vi "View one AI param scada1.vi"(5 "Sensors refs":refnum<vi>[](array[refnum]), 6 "OPC UA.Client refnum":T2, 7 "AI Descr":string[][](array[string]), 8 "error in (no error)":errorcluster, 9 "AIP":dbl[][](array[numeric]), 10 "AI_State":T3[](array[typedef]), 11 "AITable":dbl[](array[numeric]) format="%#.0f") -> (0 "error out":errorcluster)   [LabVIEW 2019, in "Inputs.lvlib"]
uses:
  Inputs.lvlib
  Ctl/Parameter State.ctl
  <vilib>/OPCUA/controls/OPC UA Client Refnum.ctl
  Ctl/View one AI param State.ctl
  <vilib>/Utility/miscctls.llb/LVRowAndColumnUnsignedTypeDef.ctl
  Ctl/AIParamColumns.ctl
  <vilib>/OPCUA/controls/NodeId.ctl
  <vilib>/OPCUA/client/Multiple Write Variant.vi
  <vilib>/OPCUA/NI OPC UA Client.lvlib
  OPC/OPC addons.lvlib
panel:
  in  "Tab Control":T1(tab)
  in  "input_register_min":dbl min=-32768.0 max=65535.0 step=1.0 format="%#.0f"
  in  "input_register_max":dbl min=-32768.0 max=65535.0 step=1.0 format="%#.0f"
  in  "input_pv_min":dbl format="%#.1f"
  in  "input_pv_max":dbl format="%#.1f"
  in  "instrument_gain":dbl min=-32768.0 max=65535.0 step=1.0 format="%#.0f"
  in  "instrument_offset":dbl format="%#.3f"
  in  "sensor num":i32
  in  "instrument_min_offset":dbl min=-32768.0 max=65535.0 step=1.0 format="%#.0f"
  in  "time_const":dbl min=-32768.0 max=65535.0 step=1.0 format="%#.0f"
  in  "fcode_full":string="кгс/см2"
  out "AI_1":dbl format="%#.1f"
  in  "Param":i32(listbox) caption="Параметры"
  in  "d":dbl min=-32768.0 max=65535.0 step=1.0 format="%#.0f"
  in  "instrument_max_offset":dbl min=-32768.0 max=65535.0 step=1.0 format="%#.0f"
  out "units":string="кгс/см2"
  in  "instrument_range_max":dbl format="%#.1f"
  in  "process_range_max":dbl format="%#.1f"
  in  "process_high_acd":dbl format="%#.1f"
  in  "process_high_alr":dbl format="%#.1f"
  in  "process_low_alr":dbl format="%#.1f"
  in  "process_low_acd":dbl format="%#.1f"
  in  "process_range_min":dbl format="%#.1f"
  in  "instrument_range_min":dbl format="%#.1f"
  # "Настройка пределов"
  # "верхнийний предел датчика"
  # "верхний предел достоверных показаний"
  # "верхний аварийный предел"
  # "верхний предупредительный предел"
  # "нижний предупредительный предел"
  # "нижний аварийный предел"
  # "нижний предел достоверных показаний"
  # "нижний предел датчика"
  # "Y"
  # "значение сигнала максимум (Ymax)"
  # "значение сигнала минимум (Ymin)"
  # "X"
  # "входной регистр минимум (Xmin)"
  # "входной регистр максимум (Xmax)"
  # "Y"
  # "массштабирование"
  # "смещение"
  # "X"
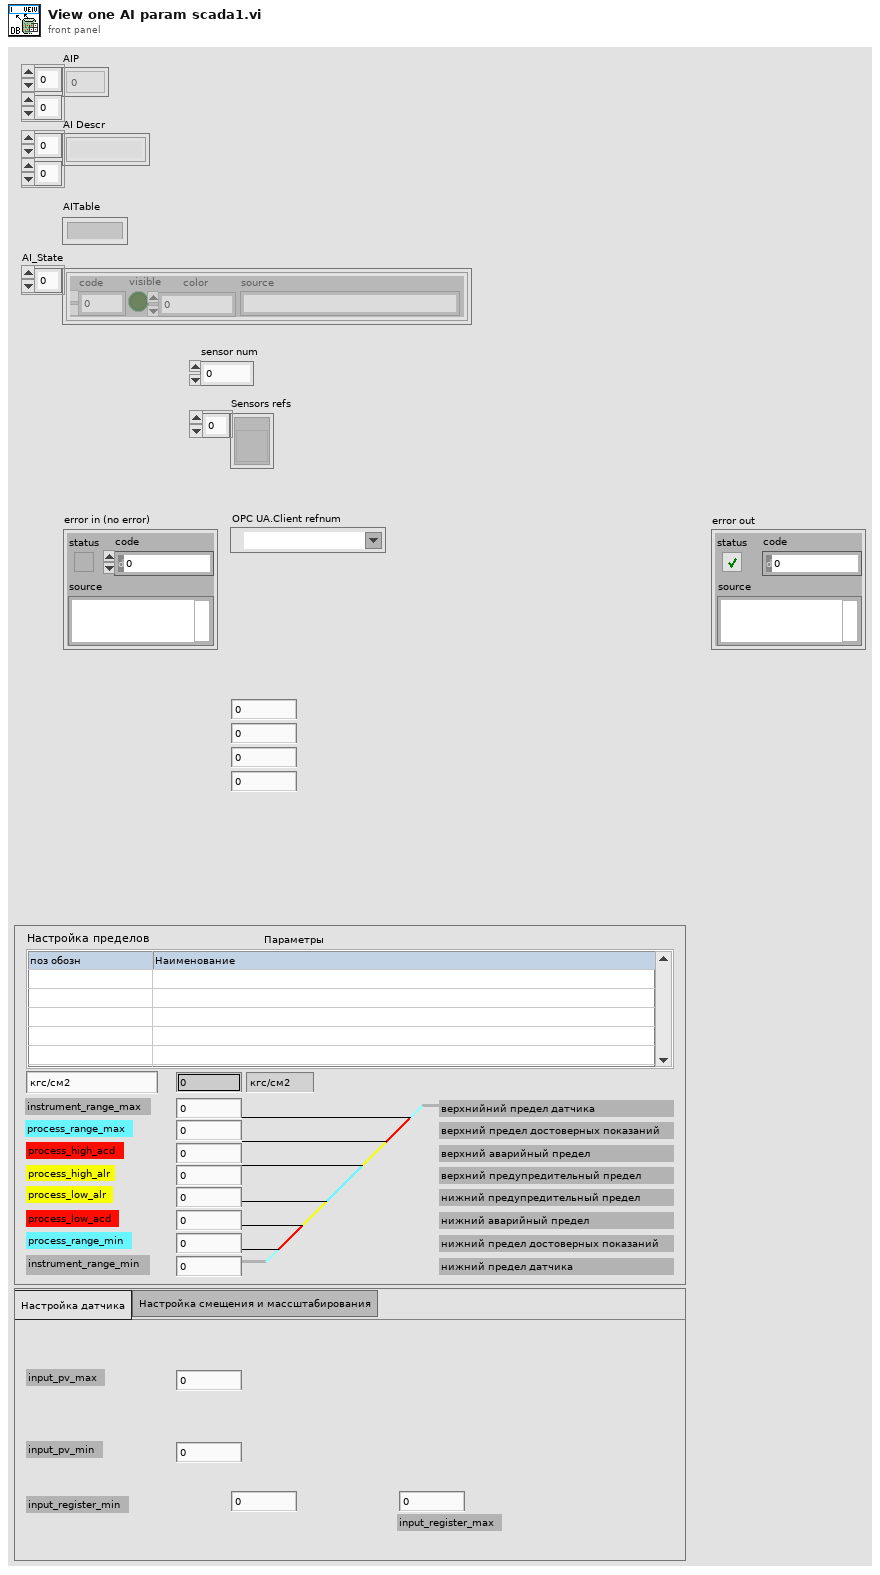
[diagram p1: front panel]
types:
  T1 = enum32{"Настройка датчика", "Настройка смещения и массштабирования"}
  T2 = typedef "OPC UA Client Refnum.ctl" = refnum<k21>
  T3 = typedef "Inputs.lvlib/Parameter State.ctl" = cluster{"code":i32, "visible":bool, "color":u32, "source":string}
  T4 = typedef "Inputs.lvlib/View one AI param State.ctl" = enum16{"init", "change sensor", "wait changes", "write parameters"}
  T5 = typedef "LVRowAndColumnUnsignedTypeDef.ctl" = cluster{"Row":u32, "Column":u32}
  T6 = typedef "NodeId.ctl" = string
  T7 = typedef "Inputs.lvlib/AIParamColumns.ctl" = enum16{"instrument_gain", "instrument_offset", "time_const", "instrument_min_offset", "instrument_range_min", "process_range_min", "process_low_acd", "process_low_alr", "process_high_alr", "process_high_acd", "process_range_max", "instrument_range_max", "instrument_max_offset", "d", "input_register_min", "input_register_max", "input_pv_min", "input_pv_max", "module_fcode_full", "control_channel_num", "ip_adress", "fcode", "fcodef", "fcode_full", "fname", "process_units"}
  T8 = typedef "Write Variant Request.ctl" = cluster{"node ID":T6, "value":variant, "timestamp (current time)":timestamp, "node status":T9}
  T9 = typedef "Write Status.ctl" = u32
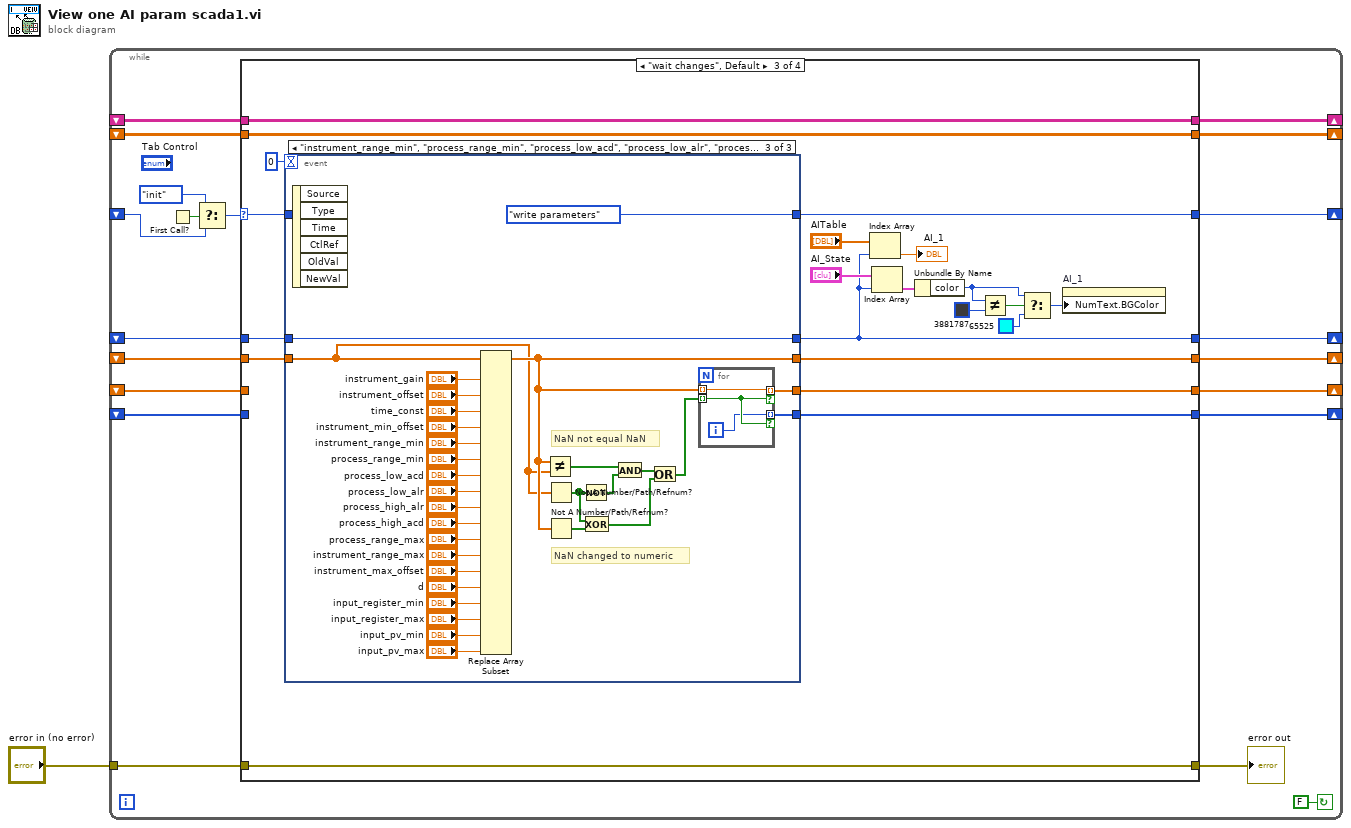
[diagram p0: block diagram]
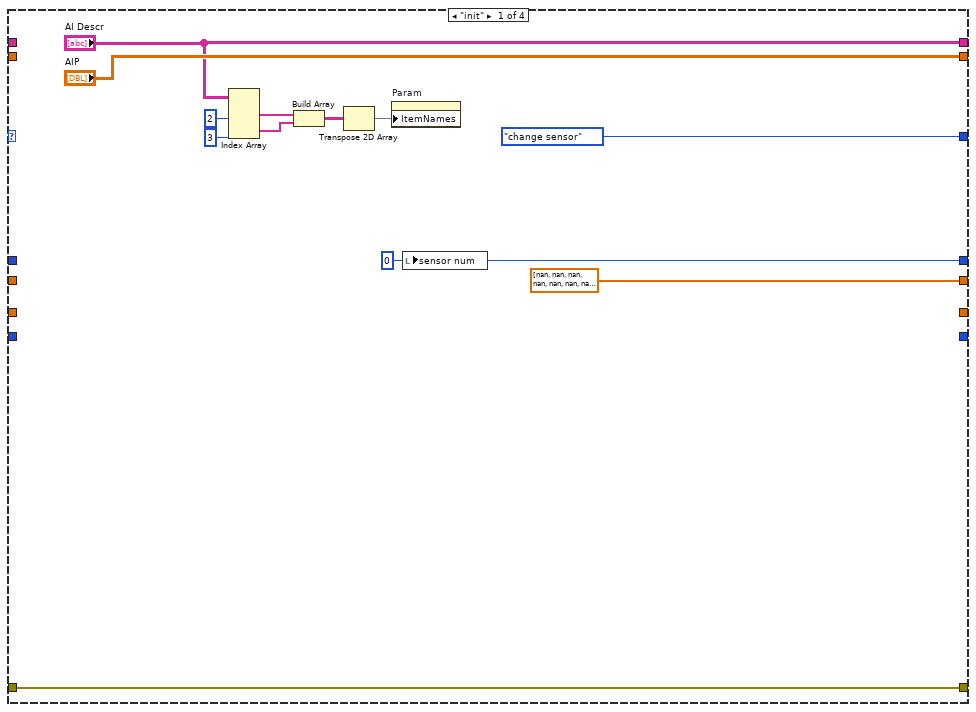
[diagram p2: hidden frame]
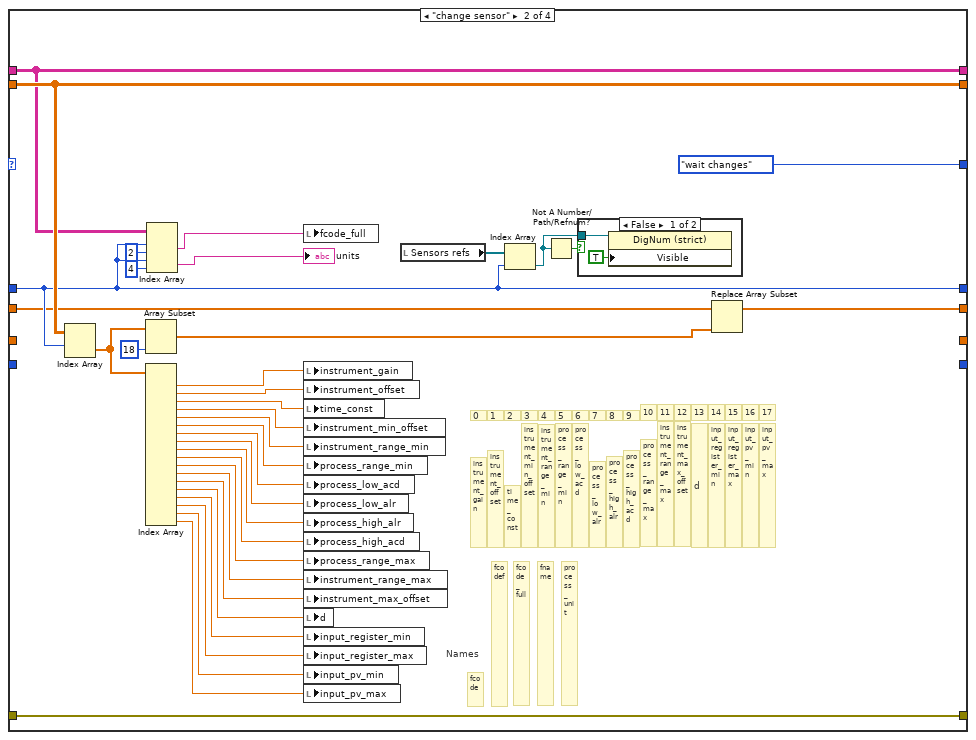
[diagram p3: hidden frame]
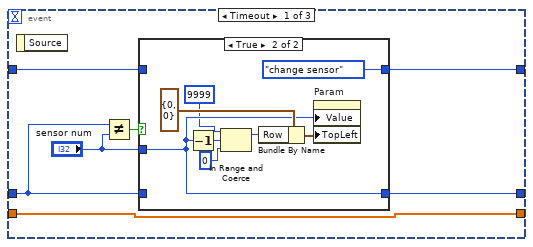
[diagram p5: hidden frame]
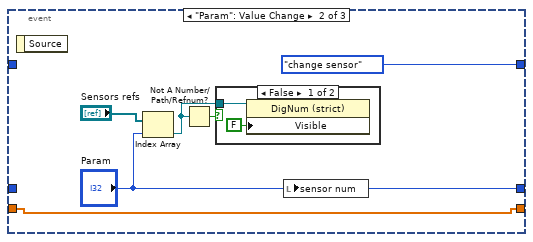
[diagram p7: hidden frame]
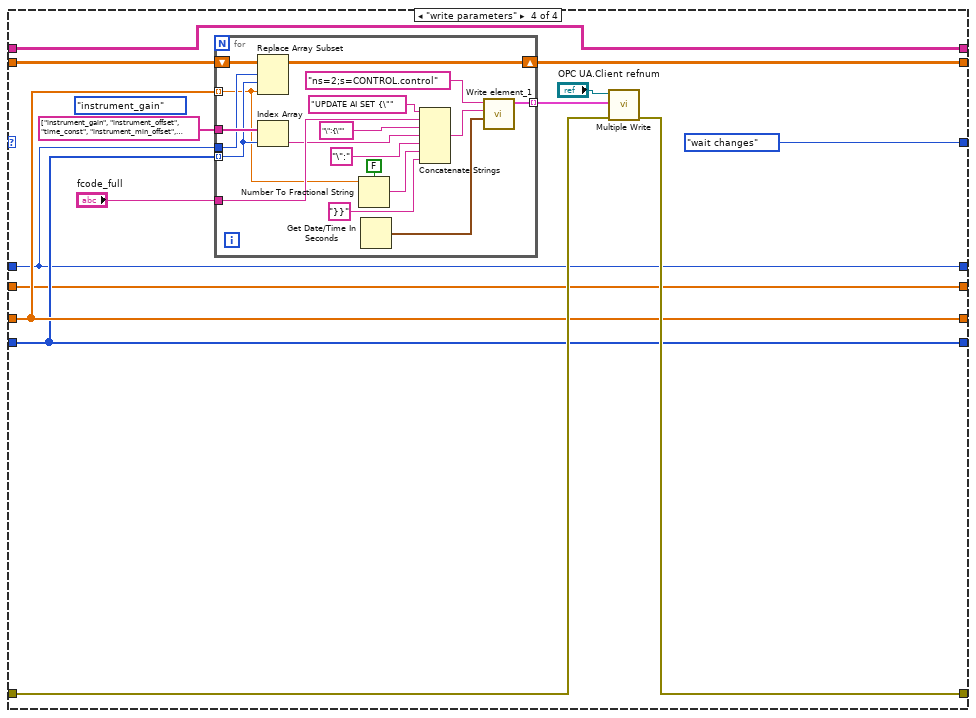
[diagram p9: hidden frame]
diagram:
  n1 = while {
    shift-right: [w19] -> _
    shift-left: _ -> [w17]
    shift-right: [w18] -> _
    shift-left: _ -> [w16]
    shift-right: [w15] -> _
    shift-left: _ -> [w14]
    tunnel: "error in (no error)" -> [w13]
    shift-right: [w12] -> _
    shift-left: _ -> [w4]
    shift-right: [w11] -> _
    shift-left: _ -> [w9]
    shift-right: [w10] -> _
    shift-left: _ -> [w8]
    shift-right: [w7] -> _
    shift-left: _ -> [w6]
    stop <- FALSE ("Boolean") continue-if-true
    n2 = First Call?() -> (First Call?: T/F=w5:bool)
    n3 = Select(t=View_one_AI_param_State."init", s=w5, f=w4) -> (s? t:f=w2:T4)
    n4 = case shown="\"wait changes\", Default" w2 {
      selector: w2 -> [_ _ w78 _]
      tunnel: w6 -> [_ w38 w76 w151]
      tunnel: w16 -> [_ w50 w87 w161]
      tunnel: w17 -> [_ w51 w86 w163]
      tunnel: [w23 w42 w85 w164] -> w21
      tunnel: [dbl[] [nan, nan, nan, nan, nan, nan, nan, nan, nan, nan, nan, nan, nan, nan, nan, nan, nan, nan] ("Parameters table") w34 w71 w152] -> w15
      tunnel: w14 -> [_ w36 w74 w152]
      tunnel: ["AIP" w51 w86 w162] -> w19
      tunnel: ["AI Descr" w50 w87 w161] -> w18
      tunnel: w13 -> [w23 w42 w85 w160]
      tunnel: [View_one_AI_param_State."change sensor" View_one_AI_param_State."wait changes" w77 View_one_AI_param_State."wait changes"] -> w12
      tunnel: [_ _ w73 w154] -> w11
      tunnel: [_ _ w72 w153] -> w10
      tunnel: w9 -> [_ _ _ w154]
      tunnel: w8 -> [_ _ _ w153]
      tunnel: [w26 w38 w75 w151] -> w7
      frame "init" {
        w26 = 0 ("sensor num")
        n5 = Index Array(array="AI Descr", index (col) #1=2 ("index (row)"), index (col) #2=3 ("index (row)")) -> (element #1=w30:string[], element #2=w29:string[])  [unwired: 2 in]
        n6 = Build Array(w30, w29) -> (w28:string[][])
        n7 = Transpose 2D Array(2D array=w28) -> (transposed array=w27:string[][])
        n8 = property on="Param" class="MCListbox (strict)"("ItemNames"=w27) -> ()  [unwired: 2 in, 2 out]
        n9 = local write "sensor num"(w26) -> ()
      }
      frame "change sensor" {
        # "fcodef"
        # "process_unit"
        # "fname"
        # "fcode_full"
        # "fcode"
        # "Names"
        # "input_pv_max"
        # "input_pv_min"
        # "input_register_max"
        # "input_register_min"
        # "d"
        # "instrument_max_offset"
        # "instrument_range_max"
        # "process_range_max"
        # "process_high_acd"
        # "process_high_alr"
        # "process_low_alr"
        # "process_low_acd"
        # "process_range_min"
        # "instrument_range_min"
        # "instrument_min_offset"
        # "time_const"
        # "instrument_gain"
        # "instrument_offset"
        # "17"
        # "16"
        # "15"
        # "14"
        # "13"
        # "12"
        # "11"
        # "10"
        # "9"
        # "8"
        # "7"
        # "6"
        # "5"
        # "4"
        # "3"
        # "2"
        # "0"
        # "1"
        n10 = Index Array(array=w51, index (row)=w38) -> (element=w53:dbl[])  [unwired: 1 in]
        n11 = Array Subset(array=w53, length=18) -> (w35:dbl[])  [unwired: 1 in]
        n12 = Index Array(array=w53) -> (element #1=w44:dbl, element #2=w45:dbl, element #3=w46:dbl, element #4=w47:dbl, element #5=w67:dbl, element #6=w66:dbl, element #7=w65:dbl, element #8=w64:dbl, element #9=w63:dbl, element #10=w62:dbl, element #11=w61:dbl, element #12=w60:dbl, element #13=w55:dbl, element #14=w54:dbl, element #15=w59:dbl, element #16=w58:dbl, element #17=w57:dbl, element #18=w56:dbl)  [unwired: 18 in]
        n13 = Index Array(array=w50, index (row) #1=w38, index (col) #1=2 ("length"), index (row) #2=w38, index (col) #2=4 ("length")) -> (element #1=w43:string, element #2=→"units":string)
        n14 = local write "fcode_full"(w43) -> ()
        n15 = local write "instrument_gain"(w44) -> ()
        n16 = local write "instrument_offset"(w45) -> ()
        n17 = local write "time_const"(w46) -> ()
        n18 = local write "instrument_min_offset"(w47) -> ()
        n19 = local write "instrument_range_min"(w67) -> ()
        n20 = local write "process_range_min"(w66) -> ()
        n21 = local write "process_low_acd"(w65) -> ()
        n22 = local write "process_low_alr"(w64) -> ()
        n23 = local write "process_high_alr"(w63) -> ()
        n24 = local write "process_high_acd"(w62) -> ()
        n25 = local write "process_range_max"(w61) -> ()
        n26 = local write "instrument_range_max"(w60) -> ()
        n27 = local write "instrument_max_offset"(w55) -> ()
        n28 = local write "d"(w54) -> ()
        n29 = local write "input_register_min"(w59) -> ()
        n30 = local write "input_register_max"(w58) -> ()
        n31 = local write "input_pv_min"(w57) -> ()
        n32 = local write "input_pv_max"(w56) -> ()
        n33 = local read "Sensors refs"() -> (w37:refnum<vi>[])
        n34 = Index Array(array=w37, index=w38) -> (element=w39:refnum<vi>)
        n35 = Not A Number/Path/Refnum?(number/path/refnum=w39) -> (NaN/Path/Refnum?=w40:bool)
        n36 = case shown="False" w40 {
          tunnel: w39 -> [w70 _]
          frame False {
            n37 = property on="Property Node" class="DigNum (strict)"(reference=w70, "Visible"=TRUE ("Blinking")) -> ()  [unwired: 1 in, 2 out]
          }
          frame True {
          }
        }
        n38 = Replace Array Subset(array=w36, new element=w35) -> (w34:dbl[])  [unwired: 1 in]
      }
      frame "wait changes", Default {
        n39 = event shown="[2] \"instrument_range_min\", \"process_range_min\", \"process_low_acd\", \"process_low_alr\", \"process_high_alr\", \"process_high_acd\", \"process_range_max\", \"instrument_range_max\", \"units\", \"input_register_min\", \"input_register_max\", \"input_pv_min\", \"input_pv_max\", \"instrument_max_offset\", \"d\", \"instrument_gain\", \"instrument_offset\": Value Change" {
          selector: _ -> [_ _ _]
          dyn-events: _ -> [_ _ _]
          timeout: 0 -> [_ _ _]
          tunnel: [w94 View_one_AI_param_State."change sensor" View_one_AI_param_State."write parameters"] -> w77
          tunnel: w78 -> [w93 _ _]
          tunnel: w76 -> [w95 _ w147]
          tunnel: [w98 "Param" w147] -> w75
          tunnel: w74 -> [w92 w109 w117]
          tunnel: [_ _ w121] -> w73
          tunnel: [_ _ w120] -> w72
          tunnel: [w92 w109 w119] -> w71
          event Timeout {
            n40 = event-data() -> ()  [unwired: 1 in, 1 out]
            n41 = Not Equal?(x=w95, y="sensor num") -> (x != y?=w97:bool)
            n42 = case shown="True" w97 {
              tunnel: "sensor num" -> [_ w104]
              tunnel: [w100 w104] -> w98
              tunnel: w95 -> [w100 _]
              tunnel: [w99 View_one_AI_param_State."change sensor"] -> w94
              tunnel: w93 -> [w99 _]
              frame False {
              }
              frame True {
                n43 = Decrement(x=w104) -> (x-1=w105:i32)
                n44 = In Range and Coerce(upper limit=9999, x=w105, lower limit=0) -> (coerced(x)=w106:i32)  [unwired: 1 out]
                n45 = Bundle By Name(cluster=T5 {"Row"=0, "Column"=0} ("Top Left Visible Cell"), "Row"=w106) -> (w107:T5)
                n46 = property on="Param" class="MCListbox (strict)"("Value"=w104, "TopLeft"=w107) -> ()  [unwired: 2 in, 2 out]
              }
            }
          }
          event "Param": Value Change {
            n47 = event-data() -> ()  [unwired: 1 in, 1 out]
            n48 = Index Array(array="Sensors refs", index="Param") -> (element=w110:refnum<vi>)
            n49 = Not A Number/Path/Refnum?(number/path/refnum=w110) -> (NaN/Path/Refnum?=w111:bool)
            n50 = case shown="False" w111 {
              tunnel: w110 -> [w116 _]
              frame False {
                n51 = property on="Property Node" class="DigNum (strict)"(reference=w116, "Visible"=FALSE ("Blinking")) -> ()  [unwired: 1 in, 2 out]
              }
              frame True {
              }
            }
            n52 = local write "sensor num"("Param") -> ()
          }
          event "instrument_range_min", "process_range_min", "process_low_acd", "process_low_alr", "process_high_alr", "process_high_acd", "process_range_max", "instrument_range_max", "units", "input_register_min", "input_register_max", "input_pv_min", "input_pv_max", "instrument_max_offset", "d", "instrument_gain", "instrument_offset": Value Change {
            # "NaN changed to numeric"
            # "NaN not equal NaN"
            n53 = event-data() -> ()  [unwired: 1 in, 6 out]
            n54 = Replace Array Subset(array=w117, new element #1="instrument_gain", new element #2="instrument_offset", new element #3="time_const", new element #4="instrument_min_offset", new element #5="instrument_range_min", new element #6="process_range_min", new element #7="process_low_acd", new element #8="process_low_alr", new element #9="process_high_alr", new element #10="process_high_acd", new element #11="process_range_max", new element #12="instrument_range_max", new element #13="instrument_max_offset", new element #14="d", new element #15="input_register_min", new element #16="input_register_max", new element #17="input_pv_min", new element #18="input_pv_max") -> (w119:dbl[])  [unwired: 18 in]
            n55 = Not Equal?(x=w119, y=w117) -> (x != y?=w136:bool[])
            n56 = Not A Number/Path/Refnum?(number/path/refnum=w117) -> (NaN/Path/Refnum?=w140:bool[])
            n57 = Not A Number/Path/Refnum?(number/path/refnum=w119) -> (NaN/Path/Refnum?=w141:bool[])
            n58 = Not(x=w140) -> (.not. x?=w139:bool[])
            n59 = Exclusive Or(1:w141, 2:w140) -> (0:w137:bool[])
            n60 = And(x=w136, y=w139) -> (x .and. y?=w138:bool[])
            n61 = Or(x=w138, y=w137) -> (x .or. y?=w135:bool[])
            n62 = for {
              tunnel: w119 -> [w150] mode=indexing
              tunnel: w135 -> [w149] mode=indexing
              tunnel: [w150] -> w121 mode=indexing if=w149
              tunnel: [w148] -> w120 mode=indexing if=w149
              i -> [w148]
            }
          }
        }
        n63 = Index Array(array="AITable", index=w75) -> (element=→"AI_1":dbl)
        n64 = Index Array(array="AI_State", index=w75) -> (element=w88:T3)
        n65 = Unbundle By Name(w88) -> ("color"=w82:u32)
        n66 = Not Equal?(x=w82, y=u32 3881787 ("color")) -> (x != y?=w83:bool)
        n67 = Select(t=w82, s=w83, f=u32 65525 ("color")) -> (s? t:f=w81:u32)
        n68 = property on="AI_1" class="DigNum (strict)"("NumText.BGColor"=w81) -> ()  [unwired: 2 in, 2 out]
      }
      frame "write parameters" {
        (unwired) AIParamColumns."instrument_gain" ("AIParamColumns")
        n69 = for {
          tunnel: w151 -> [w179]
          tunnel: string[] ["instrument_gain", "instrument_offset", "time_const", "instrument_min_offset", "instrument_range_min", "process_range_min", "process_low_acd", "process_low_alr", "process_high_alr", "process_high_acd", "process_range_max", "instrument_range_max", "instrument_max_offset", "d", "input_register_min", "input_register_max", "input_pv_min", "input_pv_max", "fcode", "fcodef", "fcode_full", "fname", "process_units"] ("AIParamColumns") -> [w182]
          tunnel: w153 -> [w176] mode=indexing
          tunnel: w154 -> [w167] mode=indexing
          shift-right: [w180] -> w162
          shift-left: w163 -> [w181]
          tunnel: "fcode_full" -> [w169]
          tunnel: [w165] -> w157 mode=indexing
          n70 = Replace Array Subset(array=w181, new element=w167, index (row)=w179, index (col)=w176) -> (w180:dbl[][])
          n71 = Index Array(array=w182, index=w176) -> (element=w168:string)
          n72 = Number To Fractional String(use system decimal point (T)=FALSE, number=w167) -> (F-format string=w175:string)  [unwired: 2 in]
          n73 = Get Date/Time In Seconds() -> (seconds since 1Jan1904=w177:timestamp)
          n74 = Concatenate Strings("UPDATE AI SET {\"" ("string"), w169, "\":{\"" ("string"), w168, "\":" ("string"), w175, "}}" ("string")) -> (w166:string)
          n75 = call "Write element_1.vi"("seconds since 1Jan1904"=w177, "Variant"=w166, "node ID"=T6 "ns=2;s=CONTROL.control") -> ("request out"=w165:T8)  [unwired: 8 in]
        }
        n76 = call-poly <vilib>:"Multiple Write.vi"("error in (no error)"=w160, "requests"=w157, "OPC UA client refnum in"="OPC UA.Client refnum") -> ("error out"=w164:errorcluster)  [unwired: 5 in, 3 out]
      }
    }
    "error out" <- w21
  }
